vi "Send cmd and wait for keywords.vi"(6 "VISA resource name":refnum<visa-resource-name>, 7 "Timeout (mSecs)":u32=3000, 8 "error in (no error)":errorcluster, 9 "Wait after":u32=750, 10 "Wait for keywords":string[](array[string]), 11 "write buffer":string) -> (0 "error out":errorcluster, 1 "Keyword found index":i32, 2 "Response":string, 3 "timeout":bool, 4 "VISA Refnum out":refnum<visa-resource-name>)   [LabVIEW 2024]
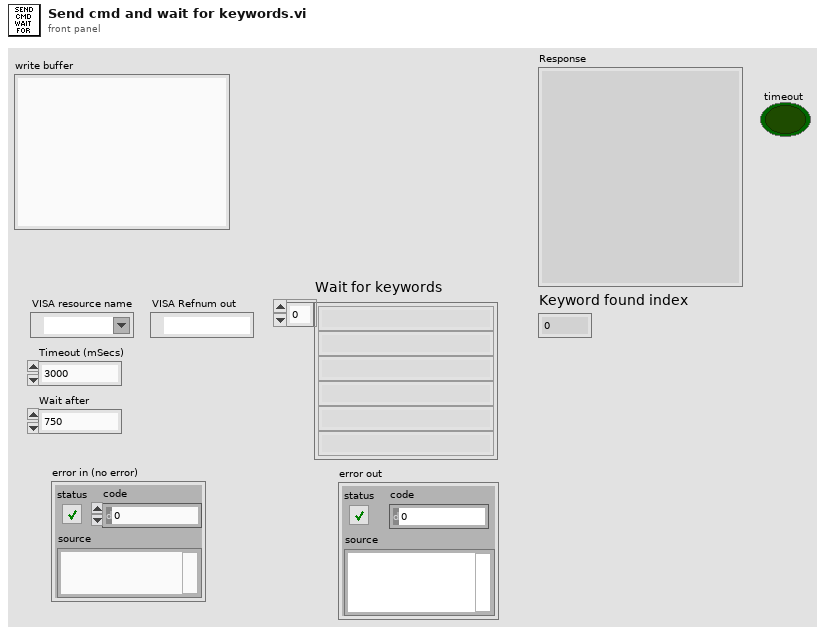
[diagram p1: front panel]
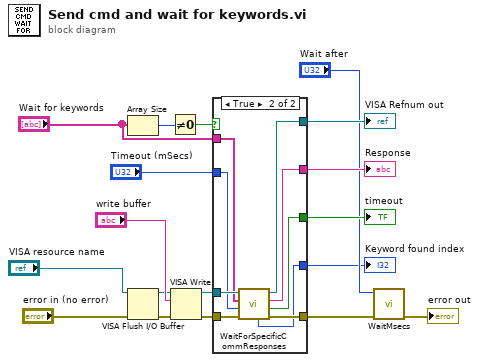
[diagram p0: block diagram]
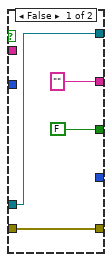
[diagram p2: hidden frame]
diagram:
  n1 = Array Size(array="Wait for keywords") -> (size(s)=w8:i32)
  n2 = VISA Flush I/O Buffer(VISA resource name="VISA resource name", error in (no error)="error in (no error)") -> (VISA resource name out=w1:refnum<visa-resource-name>, error out=w2:errorcluster)  [unwired: 1 in]
  n3 = Not Equal To 0?(x=w8) -> (x != 0?=w7:bool)
  n4 = VISA Write(VISA resource name=w1, write buffer="write buffer", error in (no error)=w2) -> (VISA resource name out=w17:refnum<visa-resource-name>, error out=w16:errorcluster)  [unwired: 1 out]
  n5 = case shown="True" w7 {
    tunnel: w17 -> [w22 w31]
    tunnel: w16 -> [w19 w30]
    tunnel: "Timeout (mSecs)" -> [_ w29]
    tunnel: ["" ("Response") w28] -> w14
    tunnel: [FALSE ("timeout") w27] -> w13
    tunnel: [w22 w26] -> w12
    tunnel: [w19 w25] -> w11
    tunnel: "Wait for keywords" -> [_ w24]
    tunnel: [_ w23] -> w5
    frame False {
    }
    frame True {
      n6 = call "WaitForSpecificCommResponses.vi"("error in (no error)"=w30, "Timeout (mSecs)"=w29, "WaitFor Keywords"=w24, "VISA Refnum in"=w31) -> ("error out"=w25:errorcluster, "timeout"=w27:bool, "Response"=w28:string, "VISA Refnum out"=w26:refnum<visa-resource-name>, "Keyword found index"=w23:i32)  [unwired: 2 in, 1 out]
    }
  }
  "VISA Refnum out" <- w12
  "Response" <- w14
  "timeout" <- w13
  "Keyword found index" <- w5
  n7 = call "WaitMsecs.vi"("error in (no error)"=w11, "Wait Msecs"="Wait after") -> ("error out"=→"error out":errorcluster)  [unwired: 9 in]
